vi "Drive Get.vi"(1 "Slow Drive?- In":bool, 2 "Axis - Y In":dbl, 3 "Axis - X In":dbl) -> (0 "Drive Info Out":T1)   [LabVIEW 2013]
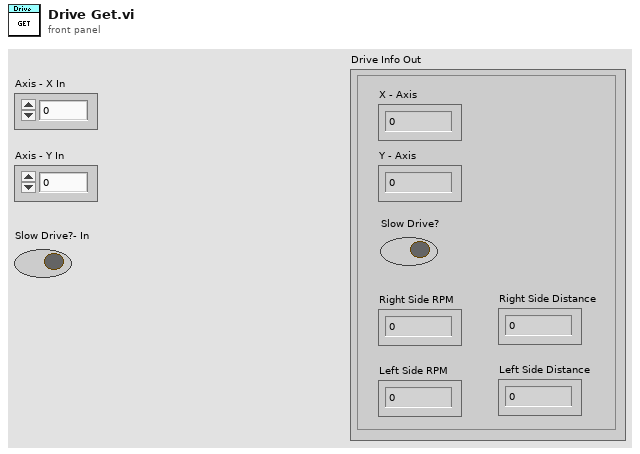
[diagram p1: front panel]
types:
  T1 = cluster{"X - Axis":dbl, "Y - Axis":dbl, "Slow Drive?":bool, "Right Side RPM":dbl, "Right Side Distance":dbl, "Left Side RPM ":dbl, "Left Side Distance":dbl}
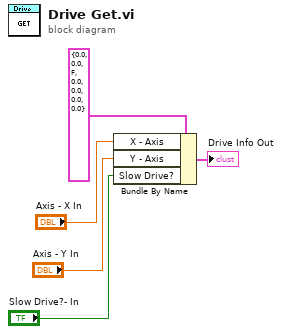
[diagram p0: block diagram]
diagram:
  n1 = Bundle By Name(cluster=T1 {"X - Axis"=0.0, "Y - Axis"=0.0, "Slow Drive?"=FALSE, "Right Side RPM"=0.0, "Right Side Distance"=0.0, "Left Side RPM "=0.0, "Left Side Distance"=0.0} ("Drive Info Out"), "X - Axis"="Axis - X In", "Y - Axis"="Axis - Y In", "Slow Drive?"="Slow Drive?- In") -> (→"Drive Info Out":T1)
